vi "Assert True.vi"(6 "error code (1)":i32=1, 7 "message":string, 8 "error in (no error)":errorcluster, 11 "True?":bool) -> (0 "error out":errorcluster)   [LabVIEW 2009]
uses:
  lvlib/Pink Elephant/Pink Elephant.lvlib
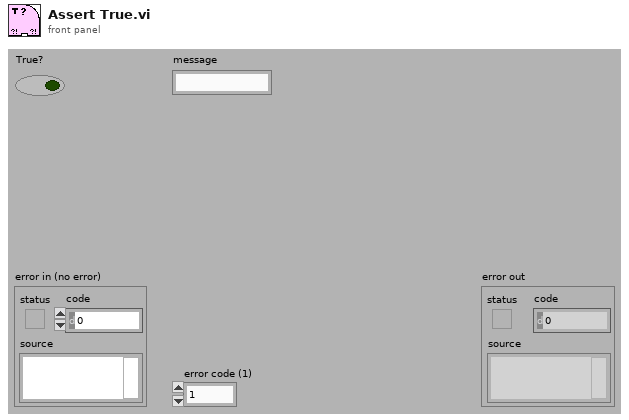
[diagram p1: front panel]
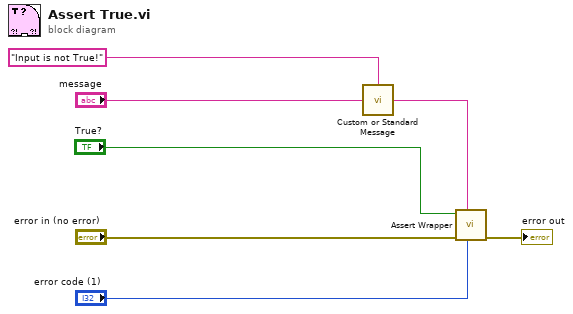
[diagram p0: block diagram]
diagram:
  n1 = call "Custom or Standard Message.vi"("Custom Message"="message", "Standard Message"="Input is not True!") -> ("Message"=w3:string)
  n2 = call "Assert Wrapper.vi"("error code (1)"="error code (1)", "Message"=w3, "error in (no error)"="error in (no error)", "Assert?"="True?") -> ("error out"=→"error out":errorcluster)  [unwired: 7 in]
